vi "Funcion_Cierre.vi"() -> ()   [LabVIEW 2016]
uses:
  mpusbapi.dll
panel:
  out "Cierre":bool
  in  "PIPE OUT":i32
  in  "PIPE IN":i32
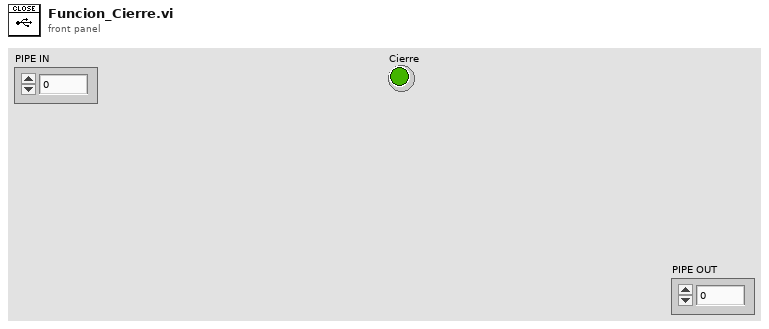
[diagram p1: front panel]
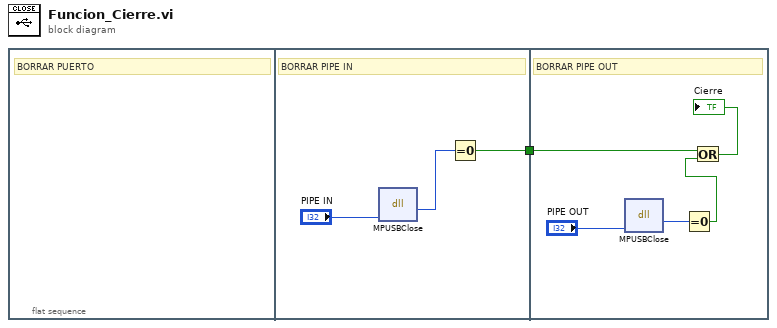
[diagram p0: block diagram]
diagram:
  n1 = flat-sequence {
    tunnel: [w2] -> w1
    tunnel: w1 -> [w6]
    frame #0 {
      # "BORRAR PUERTO"
    }
    frame #1 {
      # "BORRAR PIPE IN"
      n2 = dll-call lib="C:/microchip_solutions_v2013-06-15/USB/Tools/MCHPUSB Custom Driver/Mpusbapi/Dll/Borland_C/mpusbapi.dll" fn="MPUSBClose"("HANDLE"="PIPE IN") -> ("CIERRE"=w3:i32)  [unwired: 4 in, 2 out]
      n3 = Equal To 0?(x=w3) -> (x = 0?=w2:bool)
    }
    frame #2 {
      # "BORRAR PIPE OUT"
      n4 = dll-call lib="C:/microchip_solutions_v2013-06-15/USB/Tools/MCHPUSB Custom Driver/Mpusbapi/Dll/Borland_C/mpusbapi.dll" fn="MPUSBClose"("HANDLE"="PIPE OUT") -> ("CIERRE"=w8:i32)  [unwired: 4 in, 2 out]
      n5 = Equal To 0?(x=w8) -> (x = 0?=w7:bool)
      n6 = Or(x=w6, y=w7) -> (x .or. y?=→"Cierre":bool)
    }
  }
